vi "Check Loop Error.vi"(6 "Exit on Error? (F)":bool, 9 "Ignore Errors":i32[](array[numeric]), 10 "error to process":errorcluster, 11 "Message Queue":refnum<queue>) -> (2 "Error?":bool, 3 "dup Message Queue":refnum<queue>)   [LabVIEW 2026]
doc: "Check the 'error to process' to see if its code value matches any of the values in the 'Ignore Errors' array. If so, do nothing. If not, send an \"Error\" message containing the error data to the Message Handling Loop for further processing. If the \"Exit on Error?\" input is TRUE, send an \"Exit\" message to the Message Handling Loop instead."
uses:
  Message Queue/Message Cluster.ctl
  Message Queue/Enqueue Message (Single).vi
  Message Queue/Message Queue.lvlib
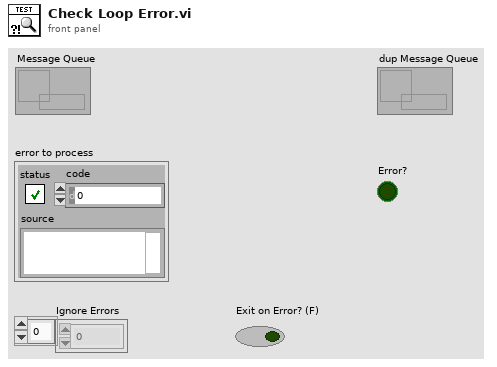
[diagram p1: front panel]
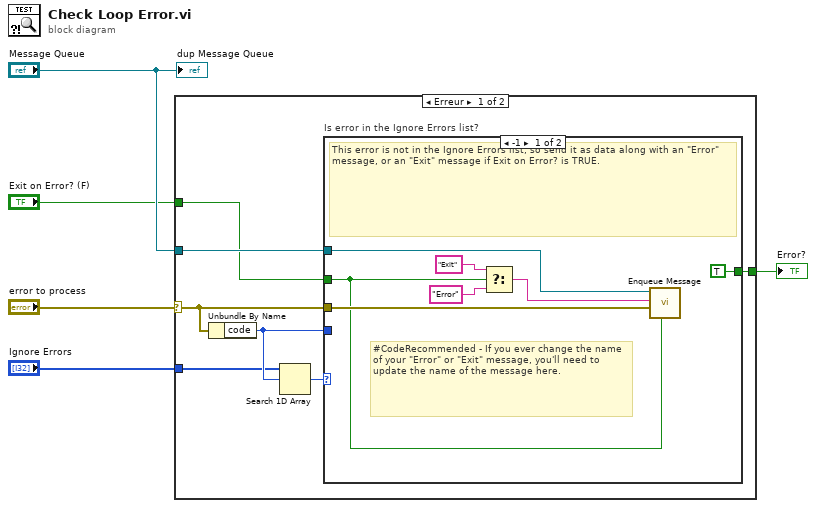
[diagram p0: block diagram]
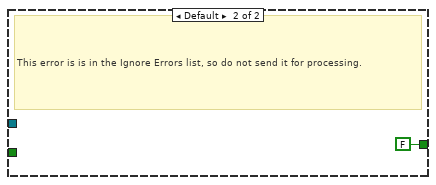
[diagram p2: hidden frame]
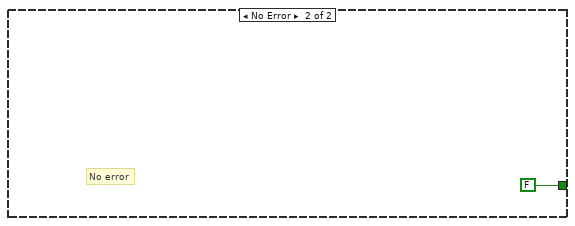
[diagram p3: hidden frame]
diagram:
  n1 = case shown="Erreur" "error to process" {
    selector: "error to process" -> [w9 _]
    tunnel: "Message Queue" -> [w12 _]
    tunnel: "Ignore Errors" -> [w8 _]
    tunnel: [w7 FALSE] -> w2
    tunnel: "Exit on Error? (F)" -> [w6 _]
    frame Error {
      n2 = Unbundle By Name(w9) -> ("code"=w10:i32)
      n3 = Search 1D Array(1D array=w8, element=w10) -> (index of element=w11:i32)  [unwired: 1 in]
      n4 = case "Is error in the Ignore Errors list?" shown="-1" w11 {
        tunnel: w9 -> [w17 _]
        tunnel: w12 -> [w19 _]
        tunnel: w10 -> [_ _]
        tunnel: [TRUE FALSE] -> w7
        tunnel: w6 -> [w16 _]
        frame -1 {
          # "#CodeRecommended - If you ever change the name of your \"Error\" or \"Exit\" message, you'll need to update the name of the message here."
          # "This error is not in the Ignore Errors list, so send it as data along with an \"Error\" message, or an \"Exit\" message if Exit on Error? is TRUE."
          n5 = Select(t="Exit" ("Message"), s=w16, f="Error" ("Message")) -> (s? t:f=w15:string)
          n6 = call-poly "Enqueue Message.vi"("Priority Message? (F)"=w16, "Message Data"=w17, "Message"=w15, "Message Queue"=w19) -> ()  [unwired: 6 in, 2 out]
        }
        frame Default {
          # "This error is is in the Ignore Errors list, so do not send it for processing."
        }
      }
    }
    frame No Error {
      # "No error"
    }
  }
  "Error?" <- w2
  "dup Message Queue" <- "Message Queue"
